vi "FPGA_Logging.vi"() -> ()   [LabVIEW 2017]
uses:
  <vilib>/rvi/Emulation/niFpgaGetClockAttributes.vi
  <vilib>/rvi/Emulation/niFpgaSctlEmulationGetInTimedLoop.vi
  <vilib>/rvi/Emulation/niFpgaEmulationReportErrorSimple.vi
  <vilib>/rvi/eio/common/nirviEmuTemplateMethod_errors.vi
  <vilib>/rvi/Emulation/niFpgaCriticalErrorInLSC.vi
  <vilib>/eio/EIONode/EIONode.xnode
panel:
  out "My Indicator":fxp<+/-,26,5> format="%.23g"
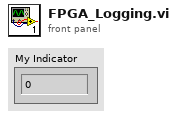
[diagram p1: front panel]
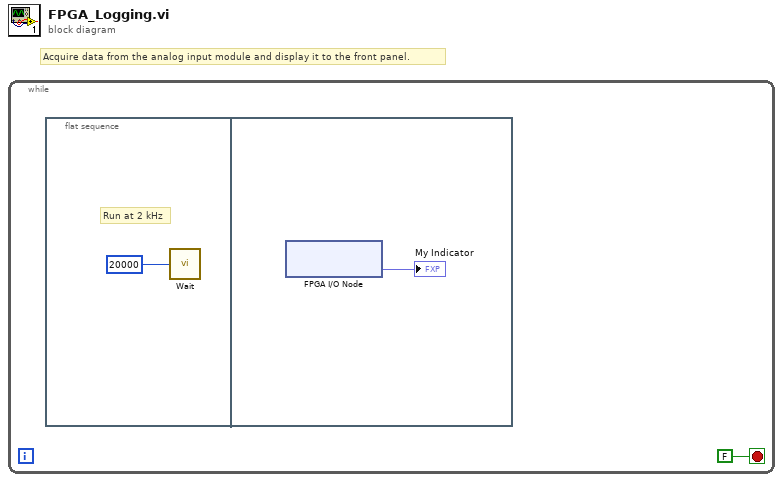
[diagram p0: block diagram]
diagram:
  # "Acquire data from the analog input module and display it to the front panel."
  n1 = while {
    stop <- FALSE stop-if-true
    n2 = flat-sequence {
      frame #0 {
        # "Run at 2 kHz"
        n3 = call "Wait"("Count(Ticks)"=u32 20000) -> ()  [unwired: 1 out]
      }
      frame #1 {
        n4 = xnode "FPGA I/O Node"() -> ("Mod3/AI0"=→"My Indicator":fxp<+/-,26,5>)  [unwired: 1 in, 1 out]
      }
    }
  }
